vi "Close.vi"(8 "error in (no error)":errorcluster, 11 "State in":T1={"State"=enum."Idle", "Start Time"=timestamp(0 s since 1904-01-01), "Configuration"={"Cycle Period"=0.0, "Mettler"={"VISA resource name"="", "Simulated?"=FALSE}, "Scale Type"=""}, "Current Time"=timestamp(0 s since 1904-01-01), "First Iteration"=FALSE, "Data"={"Scale Read(g)"=0.0}, "Process Name"="", "Log Started"=FALSE}) -> (0 "error out":errorcluster, 3 "State out":T1={"State"=enum."Idle", "Start Time"=timestamp(0 s since 1904-01-01), "Configuration"={"Cycle Period"=0.0, "Mettler"={"VISA resource name"="", "Simulated?"=FALSE}, "Scale Type"=""}, "Current Time"=timestamp(0 s since 1904-01-01), "First Iteration"=FALSE, "Data"={"Scale Read(g)"=0.0}, "Process Name"="", "Log Started"=FALSE})   [LabVIEW 2018, in "Scale Module.lvlib" / "Scale Module Engine.lvlib"]
uses:
  Scale Module Engine.lvlib
  State Cluster.ctl
  State Enum.ctl
  Feed Module/Controls/Scale Module Settings Cluster.ctl
  Mettler Toledo/Controls/Settings Cluster.ctl
  Mettler Toledo/Mettler Toledo.lvlib
  Scale Module.lvlib
panel:
  # "Scale Settings"
  # "Scale Settings"
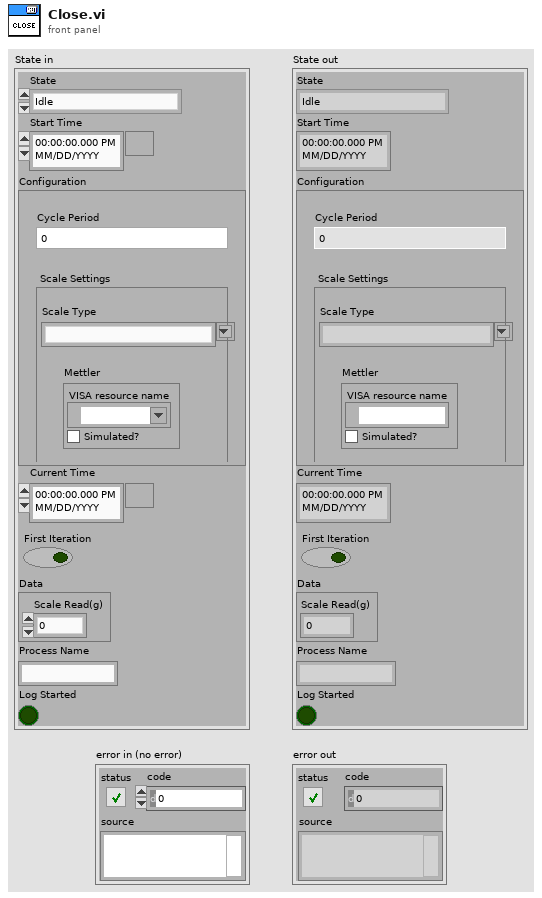
[diagram p1: front panel]
types:
  T1 = typedef "Scale Module.lvlib/Scale Module Engine.lvlib/State Cluster.ctl" = cluster{"State":T2, "Start Time":timestamp, "Configuration":T3, "Current Time":timestamp, "First Iteration":bool, "Data":cluster{"Scale Read(g)":dbl}, "Process Name":string, "Log Started":bool}
  T2 = typedef "Scale Module.lvlib/Scale Module Engine.lvlib/State Enum.ctl" = enum16{"Measuring", "Idle"}
  T3 = typedef "Scale Module.lvlib/Scale Module Settings Cluster.ctl" = cluster{"Cycle Period":dbl, "Mettler":T4, "Scale Type":string}
  T4 = typedef "Mettler Toledo.lvlib/Settings Cluster.ctl" = cluster{"VISA resource name":refnum<visa-resource-name>, "Simulated?":bool}
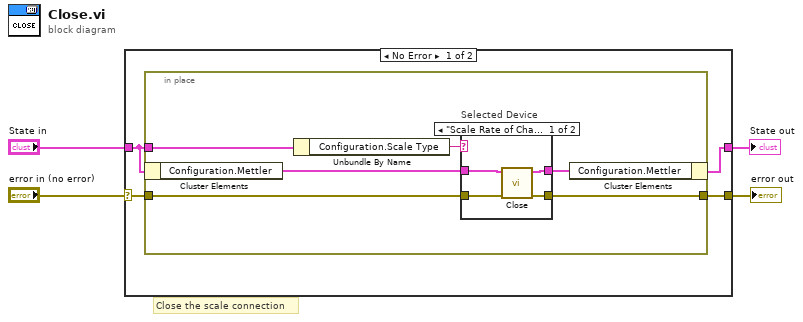
[diagram p0: block diagram]
diagram:
  # "Close the scale connection"
  n1 = case shown="No Error" "error in (no error)" {
    selector: "error in (no error)" -> [w8 w22]
    tunnel: [w7 w22] -> w3
    tunnel: "State in" -> [w6 w21]
    tunnel: [w5 w21] -> w1
    frame No Error {
      n2 = in-place {
        in-place-border: w6 -> [w13]
        in-place-border: w8 -> [w12]
        in-place-border: [w11] -> w7
        n3 = in-place-cluster #1(w6) -> ("Configuration.Mettler"=w10:T4)
        n4 = Unbundle By Name(w13) -> ("Configuration.Scale Type"=w14:string)
        n5 = case "Selected Device" shown="\"Scale Rate of Change\"" w14 {
          tunnel: w10 -> [w16 w20]
          tunnel: w12 -> [w18 w19]
          tunnel: [w17 w19] -> w11
          tunnel: [w15 w20] -> w9
          frame "Scale Rate of Change" {
            n6 = call "Close.vi"("error in (no error)"=w18, "Mettler Settings in"=w16) -> ("error out"=w17:errorcluster, "Mettler Settings out"=w15:T4)  [unwired: 8 in]
          }
          frame "Default", Default {
          }
        }
        n7 = in-place-cluster #1("Configuration.Mettler"=w9) -> (w5:T1)
      }
    }
    frame Error {
    }
  }
  "error out" <- w3
  "State out" <- w1
